vi "insert_doubles_array.vi"(8 "error in (no error)":errorcluster, 9 "Values":dbl[](array[numeric]), 10 "paths":string[](array[string]), 11 "Data.PG in":refnum<class "Data.PG.lvclass">) -> (0 "error out":errorcluster, 3 "Data.PG out":refnum<class "Data.PG.lvclass">)   [LabVIEW 2020, in "Data.PG.lvclass"]
uses:
  Data.PG.lvclass
  Data/Typedefs/Operation--enum.ctl
  Data.PG.lvclass/Data.PG.ctl
  <vilib>/JDP Science/PostgreSQL Library/Result/PQ Result.lvclass/PQ Result.ctl
  <vilib>/JDP Science/PostgreSQL Library/Connection/Execute Command (2D string results).vi
  <vilib>/JDP Science/PostgreSQL Library/Result/Clear.vi
  <vilib>/JDP Science/PostgreSQL Library/Connection/Execute Command (Result).vi
  <vilib>/JDP Science/PostgreSQL Library/Connection/Execute (Return first result with rows).vi
  <vilib>/JDP Science/PostgreSQL Library/Connection/Single Command with parameters.vi
  <vilib>/JDP Science/PostgreSQL Library/Result/Get all results as 2D strings array.vi
  <vilib>/JDP Science/PostgreSQL Library/Connection/PQ Connection.lvclass
  Data/Data.lvclass
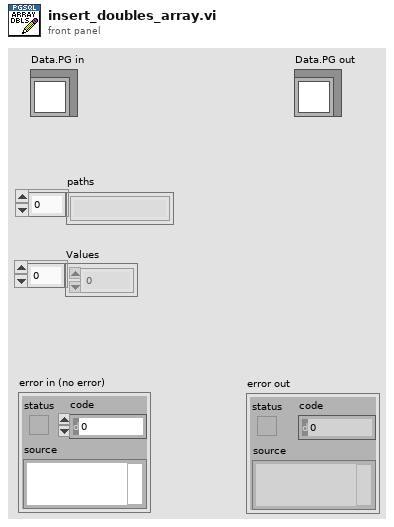
[diagram p1: front panel]
types:
  T1 = typedef "Data.lvclass/Operation--enum.ctl" = enum16{"Read", "Write", "Write + Append"}
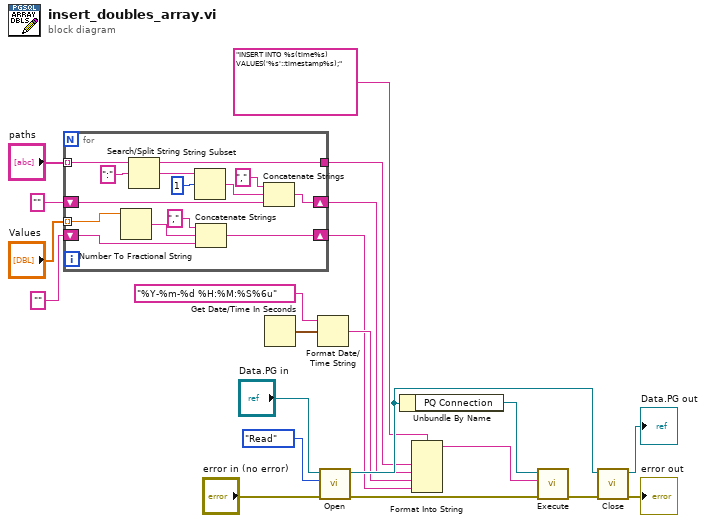
[diagram p0: block diagram]
diagram:
  n1 = for {
    tunnel: "paths" -> [w32] mode=indexing
    tunnel: "Values" -> [w26] mode=indexing
    shift-right: [w30] -> w6
    shift-left: "" -> [w29]
    tunnel: [w28] -> w7
    shift-right: [w23] -> w1
    shift-left: "" -> [w22]
    n2 = Number To Fractional String(number=w26) -> (F-format string=w25:string)  [unwired: 3 in]
    n3 = Search/Split String(string=w32, search string/char (-)=":") -> (substring before match=w28:string, match + rest of string=w34:string)  [unwired: 1 in, 1 out]
    n4 = String Subset(string=w34, offset (0)=1) -> (substring=w31:string)  [unwired: 1 in]
    n5 = Concatenate Strings("," ("string"), w25, w22) -> (w23:string)
    n6 = Concatenate Strings("," ("string"), w31, w29) -> (w30:string)
  }
  n7 = Get Date/Time In Seconds() -> (seconds since 1Jan1904=w4:timestamp)
  n8 = Format Date/Time String(time format string (%c)="%Y-%m-%d %H:%M:%S%6u", seconds (now)=w4) -> (date/time string=w3:string)  [unwired: 1 in]
  n9 = call-dynamic "Open.vi"("error in (no error)"="error in (no error)", "Operation"=Operation--enum."Read", "Data.PG in"="Data.PG in") -> ("error out"=w18:errorcluster, "Data.PG out"=w13:refnum<class "Data.PG.lvclass">)  [unwired: 7 in]
  n10 = Unbundle By Name(w13) -> ("PQ Connection"=w12:refnum<class "PQ Connection.lvclass">)
  n11 = Format Into String(format string="INSERT INTO %s(time%s) VALUES('%s'::timestamp%s);", w7, w6, w3, w1) -> (resulting string=w14:string)  [unwired: 2 in, 1 out]
  n12 = call-poly <vilib>:"Execute.vi"("error in (no error)"=w18, "SQL"=w14, "PQ Connection in"=w12) -> ("error out"=w17:errorcluster)  [unwired: 5 in, 3 out]
  n13 = call-dynamic "Close.vi"("error in (no error)"=w17, "Data.PG in"=w13) -> ("error out"=→"error out":errorcluster, "Data.PG out"=→"Data.PG out":refnum<class "Data.PG.lvclass">)  [unwired: 8 in]
